vi "daq_example_stimulate.vi"() -> ()   [LabVIEW 2015]
uses:
  <vilib>/DAQmx/write.llb/DAQmx Write (Analog Wfm 1Chan NSamp).vi
  <vilib>/DAQmx/create/channels.llb/DAQmx Create Channel (AO-Voltage-Basic).vi
  <vilib>/DAQmx/configure/timing.llb/DAQmx Timing (Sample Clock).vi
  <vilib>/DAQmx/miscellaneous.llb/DAQmx Fill In Error Info.vi
  <resource>/objmgr/daqmx.rc
panel:
  out "Actual Sample Rate":dbl=1000.0 format="%0.2f"
  out "Numeric":dbl
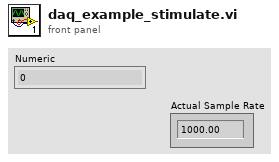
[diagram p1: front panel]
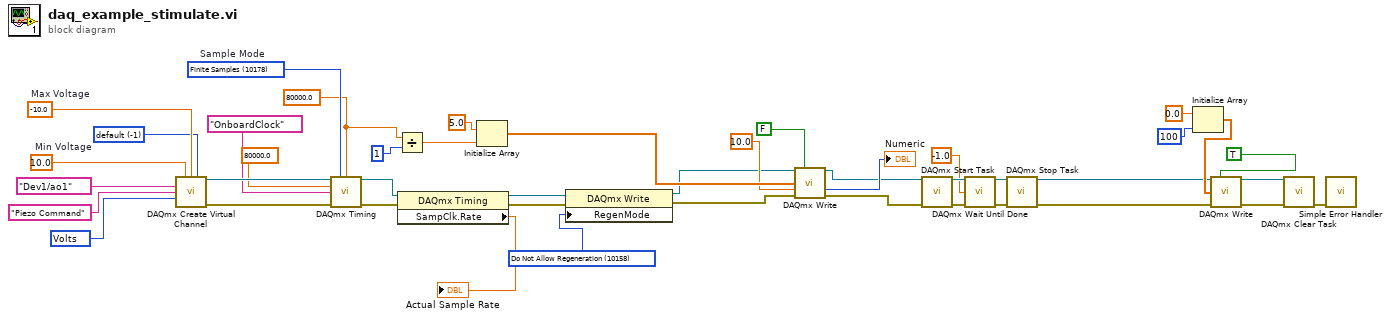
[diagram p0: block diagram]
diagram:
  w9 = 10158 items=["Allow Regeneration"=10097, "Do Not Allow Regeneration"=10158] ("RegenMode")
  w18 = 80000.0
  w34 = 10178 items=["Finite Samples"=10178, "Continuous Samples"=10123, "Hardware Timed Single Point"=12522]  # Sample Mode
  w35 = -1 items=["default"=-1, "RSE"=10083, "NRSE"=10078, "Differential"=10106, "Pseudodifferential"=12529] ("input terminal configuration")
  w36 = 10348 items=["Volts"=10348, "From Custom Scale"=10065] ("units")
  w40 = 10.0  # Min Voltage
  w39 = -10.0  # Max Voltage
  n1 = call-poly <vilib>:"DAQmx Create Virtual Channel.vi"("maximum value"=w40, "minimum value"=w39, "output terminal configuration"=w35, "physical channels"=tag "Dev1/ao1" ("DAQmx Physical Channel"), "name to assign"="Piezo Command", "units"=w36) -> ("task out"=w42:refnum<k21>, "error out"=w43:errorcluster)  [unwired: 8 in]
  n2 = call-poly <vilib>:"DAQmx Timing.vi"("task/channels in"=w42, "sample mode"=w34, "samples per channel"=w18, "rate"=80000.0, "source"=tag "OnboardClock" ("Sample Clock Source"), "error in"=w43) -> ("task out"=w32:refnum<k21>, "error out"=w31:errorcluster)  [unwired: 8 in]
  n3 = Divide(x=w18, y=1) -> (x/y=w17:dbl)
  n4 = property class="DAQmx Timing"(reference=w32, error in=w31) -> (reference out=w15:refnum<k21>, error out=w14:errorcluster, "SampClk.Rate"=→"Actual Sample Rate":dbl)
  n5 = Initialize Array(5.0 ("element"), w17) -> (w22:dbl[])
  n6 = property class="DAQmx Write"(reference=w15, error in=w14, "RegenMode"=w9) -> (reference out=w13:refnum<k21>, error out=w12:errorcluster)
  n7 = call-poly <vilib>:"DAQmx Write.vi"("task/channels in"=w13, "auto start"=FALSE, "data"=w22, "timeout"=10.0, "error in"=w12) -> ("task out"=w10:refnum<k21>, "number of samples written per channel"=→"Numeric":u32, "error out"=w11:errorcluster)  [unwired: 8 in]
  n8 = call <vilib>:"DAQmx Start Task.vi"("task/channels in"=w10, "error in"=w11) -> ("task out"=w25:refnum<k21>, "error out"=w26:errorcluster)  [unwired: 12 in]
  n9 = call <vilib>:"DAQmx Wait Until Done.vi"("task/channels in"=w25, "timeout (sec)"=-1.0, "error in"=w26) -> ("task out"=w28:refnum<k21>, "error out"=w27:errorcluster)  [unwired: 11 in]
  n10 = call <vilib>:"DAQmx Stop Task.vi"("task/channels in"=w28, "error in"=w27) -> ("task out"=w3:refnum<k21>, "error out"=w2:errorcluster)  [unwired: 12 in]
  n11 = Initialize Array(0.0 ("element"), 100 ("dimension size")) -> (w5:dbl[])
  n12 = call-poly <vilib>:"DAQmx Write.vi"("task/channels in"=w3, "auto start"=TRUE, "data"=w5, "error in"=w2) -> ("task out"=w8:refnum<k21>, "error out"=w7:errorcluster)  [unwired: 9 in, 1 out]
  n13 = call <vilib>:"DAQmx Clear Task.vi"("task in"=w8, "error in"=w7) -> ("error out"=w24:errorcluster)  [unwired: 13 in]
  n14 = call <vilib>:"Simple Error Handler.vi"("error in (no error)"=w24) -> ()  [unwired: 4 in, 5 out]
